vi "Main.vi"() -> ()   [LabVIEW 2017]
doc: "Use this template to build a simple state machine design pattern. Each state executes code and determines which state to transition to."
uses:
  controls/State.ctl
  controls/Data.ctl
panel:
  in  "Do Something Else <Replace Me>":bool
  in  "Do Something <Replace Me>":bool
  in  "Exit":bool
  # "These controls have associated \"Value Changed\" events configured in the Event Structure on the diagram.\n\nReplace them (and reconfigure the Event Structure) with the controls you need for your application."
  # "This template is for the Simple State Machine design pattern.\n\nSee the block diagram for more information on how to use this template."
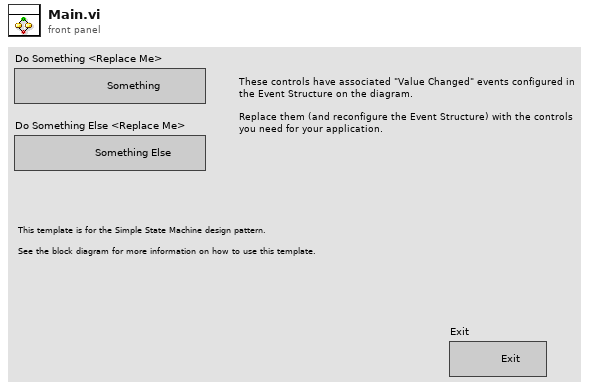
[diagram p1: front panel]
types:
  T1 = typedef "Data.ctl" = cluster{"Boolean <Replace Me>":bool, "String <Replace Me>":string, "Numeric <Replace Me>":dbl}
  T2 = typedef "State.ctl" = enum16{"Initialize", "Wait for Event", "User State 1", "User State 2", "Exit"}
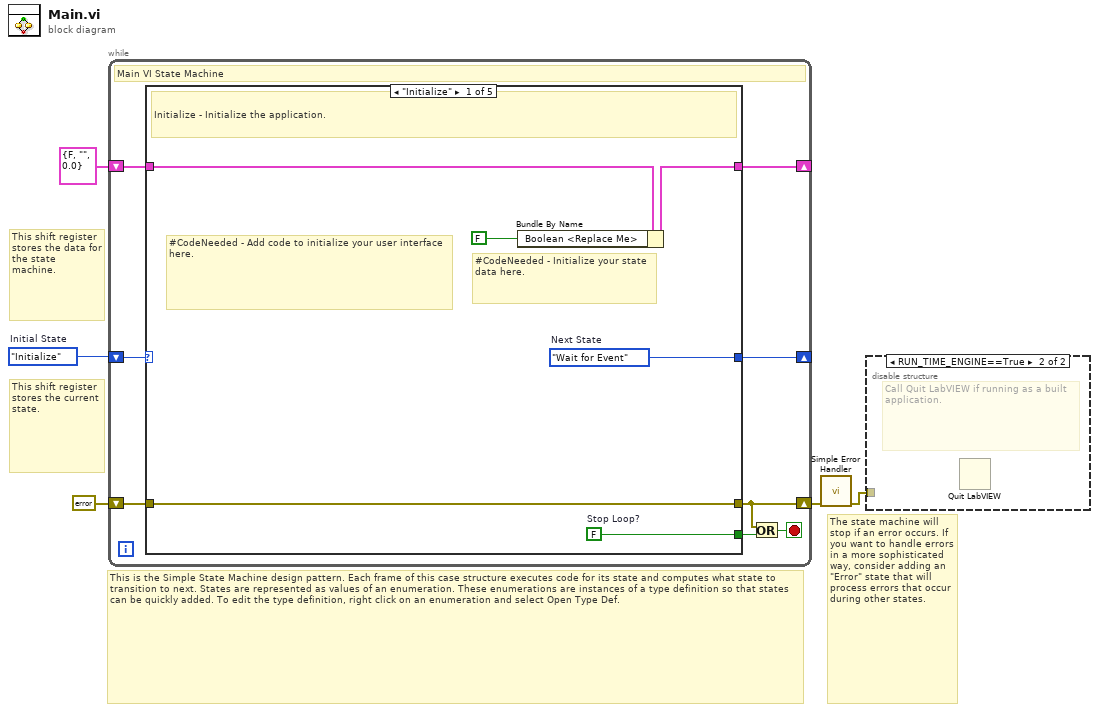
[diagram p0: block diagram]
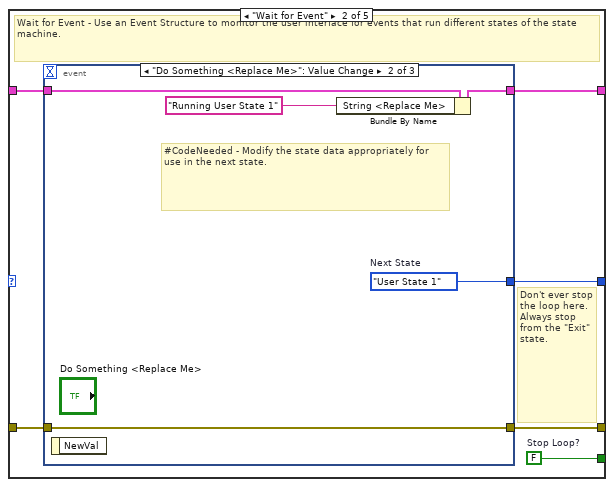
[diagram p3: hidden frame]
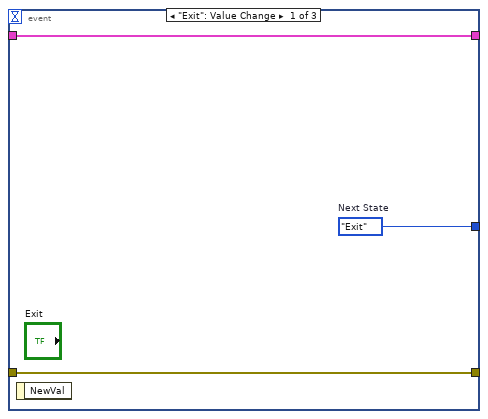
[diagram p4: hidden frame]
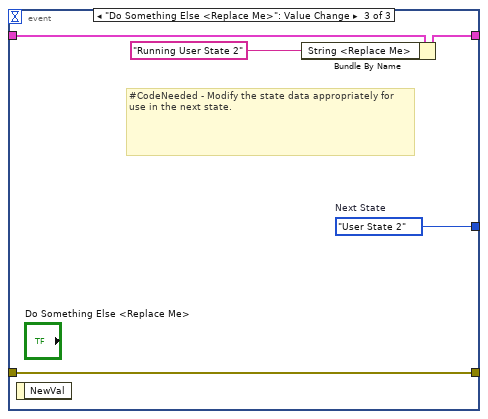
[diagram p5: hidden frame]
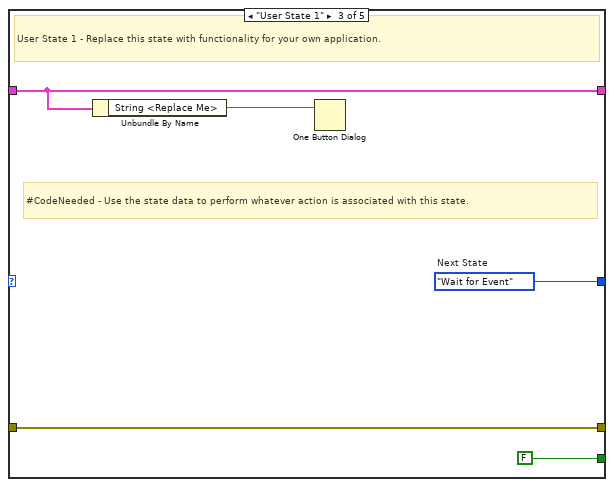
[diagram p6: hidden frame]
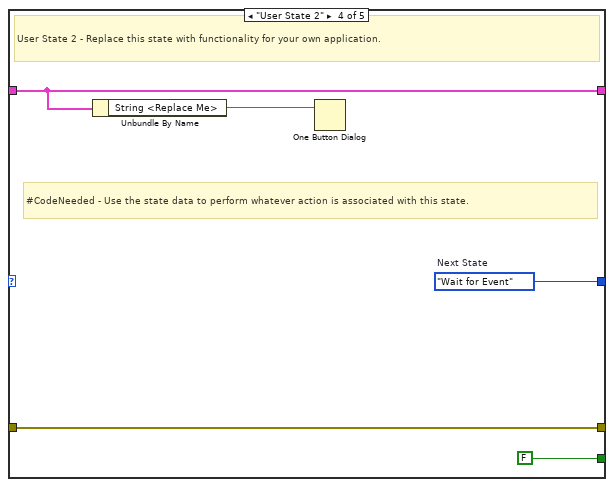
[diagram p7: hidden frame]
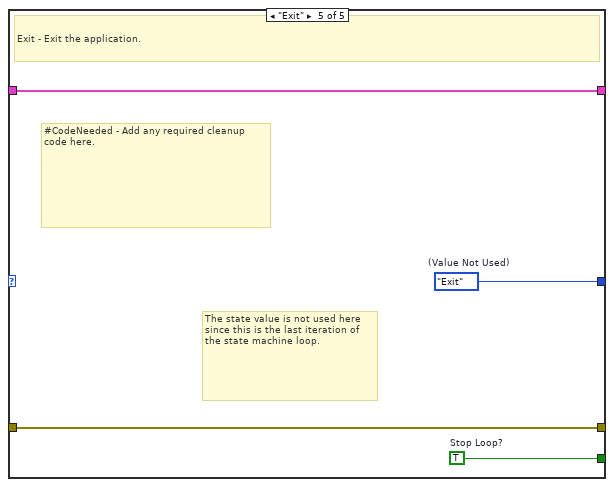
[diagram p8: hidden frame]
diagram:
  w5 = State."Initialize"  # Initial State
  # "The state machine will stop if an error occurs. If you want to handle errors in a more sophisticated way, consider adding an \"Error\" state that will process errors that occur during other states."
  # "This shift register stores the data for the state machine."
  # "This is the Simple State Machine design pattern. Each frame of this case structure executes code for its state and computes what state to transition to next. States are represented as values of an enumeration. These enumerations are instances of a type definition so that states can be quickly added. To edit the type definition, right click on an enumeration and select Open Type Def."
  # "This shift register stores the current state."
  n1 = while {
    shift-right: [w12] -> _
    shift-left: w5 -> [w13]
    shift-right: [w10] -> _
    shift-left: T1 {"Boolean <Replace Me>"=FALSE, "String <Replace Me>"="", "Numeric <Replace Me>"=0.0} ("Data") -> [w11]
    shift-right: [w6] -> w2
    shift-left: errorcluster {"status"=FALSE, "code"=0, "source"=""} ("error constant") -> [w9]
    stop <- w7 stop-if-true
    # "Main VI State Machine"
    n2 = case shown="\"Initialize\"" w13 {
      tunnel: [w19 w25 w43 w48 w52] -> w12
      tunnel: [w18 w24 FALSE ("Stop Loop?") FALSE ("Stop Loop?") w50] -> w8
      tunnel: w11 -> [w17 w23 w41 w46 w51]
      tunnel: [w16 w22 w41 w46 w51] -> w10
      tunnel: w9 -> [w14 w21 w39 w44 w49]
      tunnel: [w14 w20 w39 w44 w49] -> w6
      frame "Initialize" {
        w18 = FALSE  # Stop Loop?
        w19 = State."Wait for Event"  # Next State
        # "#CodeNeeded - Initialize your state data here."
        # "#CodeNeeded - Add code to initialize your user interface here."
        # "Initialize - Initialize the application."
        n3 = Bundle By Name(cluster=w17, "Boolean <Replace Me>"=FALSE ("Replace_Me_Boolean")) -> (w16:T1)
      }
      frame "Wait for Event" {
        w24 = FALSE  # Stop Loop?
        # "Don't ever stop the loop here. Always stop from the \"Exit\" state."
        # "Wait for Event - Use an Event Structure to monitor the user interface for events that run different states of the state machine."
        n4 = event shown="[1] \"Do Something <Replace Me>\": Value Change" {
          selector: _ -> [_ _ _]
          dyn-events: _ -> [_ _ _]
          timeout: _ -> [_ _ _]
          tunnel: [w28 w33 w38] -> w25
          tunnel: w23 -> [w27 w32 w37]
          tunnel: [w27 w31 w36] -> w22
          tunnel: w21 -> [w26 w29 w34]
          tunnel: [w26 w29 w34] -> w20
          event "Exit": Value Change {
            w28 = State."Exit"  # Next State
            n5 = event-data() -> ()  [unwired: 1 in, 1 out]
          }
          event "Do Something <Replace Me>": Value Change {
            w33 = State."User State 1"  # Next State
            # "#CodeNeeded - Modify the state data appropriately for use in the next state."
            n6 = event-data() -> ()  [unwired: 1 in, 1 out]
            n7 = Bundle By Name(cluster=w32, "String <Replace Me>"="Running User State 1" ("Running User State 1")) -> (w31:T1)
          }
          event "Do Something Else <Replace Me>": Value Change {
            w38 = State."User State 2"  # Next State
            # "#CodeNeeded - Modify the state data appropriately for use in the next state."
            n8 = event-data() -> ()  [unwired: 1 in, 1 out]
            n9 = Bundle By Name(cluster=w37, "String <Replace Me>"="Running User State 2" ("Running User State 2")) -> (w36:T1)
          }
        }
      }
      frame "User State 1" {
        w43 = State."Wait for Event"  # Next State
        # "#CodeNeeded - Use the state data to perform whatever action is associated with this state."
        # "User State 1 - Replace this state with functionality for your own application."
        n10 = Unbundle By Name(w41) -> ("String <Replace Me>"=w40:string)
        n11 = One Button Dialog(message=w40) -> ()  [unwired: 1 in, 1 out]
      }
      frame "User State 2" {
        w48 = State."Wait for Event"  # Next State
        # "#CodeNeeded - Use the state data to perform whatever action is associated with this state."
        # "User State 2 - Replace this state with functionality for your own application."
        n12 = Unbundle By Name(w46) -> ("String <Replace Me>"=w45:string)
        n13 = One Button Dialog(message=w45) -> ()  [unwired: 1 in, 1 out]
      }
      frame "Exit" {
        w50 = TRUE  # Stop Loop?
        w52 = State."Exit"  # (Value Not Used)
        # "#CodeNeeded - Add any required cleanup code here."
        # "The state value is not used here since this is the last iteration of the state machine loop."
        # "Exit - Exit the application."
      }
    }
    n14 = Or(x=w6, y=w8) -> (x .or. y?=w7:bool)
  }
  n15 = call <vilib>:"Simple Error Handler.vi"("error in (no error)"=w2) -> ("error out"=w1:errorcluster)  [unwired: 4 in, 4 out]
  n16 = disable-structure shown="RUN_TIME_ENGINE==True" {
    disable-tunnel: w1 -> [_ _]
    frame condition #0 (active) {
    }
    frame condition #1 {
      # "Call Quit LabVIEW if running as a built application."
      n17 = Quit LabVIEW() -> ()  [unwired: 1 in]
    }
  }
